vi "实验3 频率调制TX.vi"() -> ()   [LabVIEW 2015]
uses:
  <instrlib>/niUSRP/niUSRP Write Tx Data (CDB WDT).vi
panel:
  in  "同时播放？":bool
  out "错误":bool
  in  "FM频偏(Hz)":dbl=100000.0 format="%#_6p"
  in  "天线":string(combo)="TX1"
  in  "载波频率":dbl=800000000.0 format="%#_6p"
  in  "IQ 速率":dbl=400000.0 format="%#_6p"
  in  "增益":dbl format="%#_6f"
  in  "设备IP地址":refnum<k15>="192.168.10.2"
  out "FM调制信号(时域)":dbl[](graph) caption="FM 调制信号(时域)"
  out "FM调制信号(频域)":cluster{"f0":dbl, "df":dbl, "magnitude":dbl[]}(graph)={"f0"=-99993.30579988277, "df"=13.387776917911738, "magnitude"=[]}
  out "音频波形":waveform(dbl)(graph)={"t0"=timestamp(24.71655328798186 s since 1904-01-01), "dt"=2.2675736961451248e-05, "Y"=[]}
  in  "停止":bool
  in  "文件路径":path
  # "实验3 频率调制 TX"
  # "硬件参数配置"
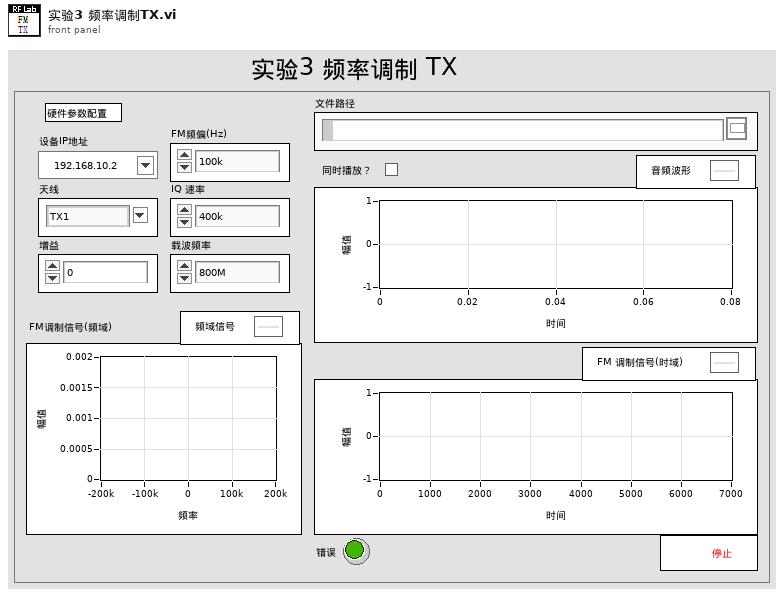
[diagram p1: front panel]
types:
  T1 = typedef "Sound Output Task ID.ctl" = u32
  T2 = typedef "Sound File Refnum.ctl" = refnum<file>
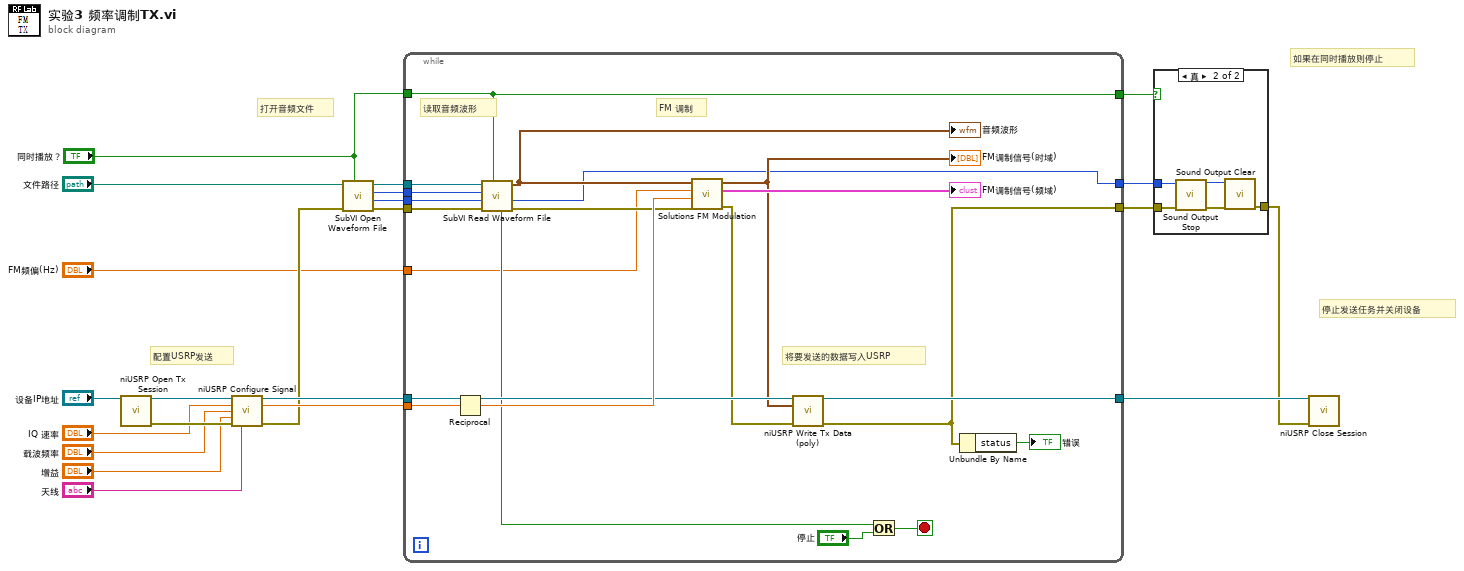
[diagram p0: block diagram]
diagram:
  # "停止发送任务并关闭设备"
  # "如果在同时播放则停止"
  # "配置USRP发送"
  # "打开音频文件"
  n1 = call <instrlib>:"niUSRP Open Tx Session.vi"("device names"="设备IP地址") -> ("session handle out"=w10:refnum<k15>, "error out"=w9:errorcluster)  [unwired: 13 in]
  n2 = call <instrlib>:"niUSRP Configure Signal.vi"("session handle"=w10, "IQ rate"="IQ 速率", "carrier frequency"="载波频率", "gain"="增益", "error in (no error)"=w9, "active antenna"="天线") -> ("session handle out"=w20:refnum<k15>, "coerced IQ rate"=w15:dbl, "error out"=w13:errorcluster)  [unwired: 5 in, 2 out]
  n3 = call "SubVI Open Waveform File.vi"("同时播放？"="同时播放？", "错误输入"=w13, "文件路径"="文件路径") -> ("错误输出"=w17:errorcluster, "音频输出任务ID"=w16:T1, "每通道采样数"=w14:i32, "声音文件引用句柄"=w21:T2)  [unwired: 5 in]
  n4 = while {
    tunnel: w21 -> [w43]
    tunnel: w17 -> [w42]
    tunnel: w15 -> [w40]
    tunnel: w20 -> [w39]
    tunnel: [w38] -> w3
    tunnel: [w25] -> w19
    tunnel: [w31] -> w18
    tunnel: w16 -> [w29]
    tunnel: w14 -> [w28]
    tunnel: "FM频偏(Hz)" -> [w26]
    tunnel: "同时播放？" -> [w23]
    tunnel: [w23] -> w1
    stop <- w37 stop-if-true
    # "将要发送的数据写入USRP"
    # "FM 调制"
    # "读取音频波形"
    n5 = Reciprocal(x=w40) -> (1/x=w41:dbl)
    n6 = call "SubVI Read Waveform File.vi"("同时播放？"=w23, "错误输入（无错误）"=w42, "音频输出任务ID"=w29, "每通道采样数"=w28, "声音文件引用句柄"=w43) -> ("错误输出"=w34:errorcluster, "音频输出任务ID"=w31:T1, "音频数据输出"=w35:waveform(dbl), "文件结束?"=w30:bool)  [unwired: 3 in]
    "音频波形" <- w35
    n7 = call "Solutions FM Modulation.vi"("错误输入(无错误)"=w34, "采样间隔(s)"=w41, "FM 频偏(Hz)"=w26, "数据输入"=w35) -> ("错误输出"=w27:errorcluster, "FM 调制信号(频域)"=→"FM调制信号(频域)":cluster{"f0":dbl, "df":dbl, "magnitude":dbl[]}, "FM 调制信号(时域)"=w32:waveform(cdb))  [unwired: 5 in]
    "FM调制信号(时域)" <- w32
    n8 = call-poly <instrlib>:"niUSRP Write Tx Data (poly).vi"("session handle"=w39, "data"=w32, "error in (no error)"=w27) -> ("session handle out"=w38:refnum<k15>, "error out"=w25:errorcluster)  [unwired: 11 in]
    n9 = Or(x=w30, y="停止") -> (x .or. y?=w37:bool)
    n10 = Unbundle By Name(w25) -> ("status"=→"错误":bool)
  }
  n11 = case shown="真" w1 {
    tunnel: w19 -> [w44 w49]
    tunnel: w18 -> [_ w48]
    tunnel: [w44 w45] -> w2
    frame False {
    }
    frame True {
      n12 = call <vilib>:"Sound Output Stop.vi"("error in (no error)"=w49, "task ID"=w48) -> ("error out"=w47:errorcluster, "task ID out"=w46:T1)  [unwired: 8 in]
      n13 = call <vilib>:"Sound Output Clear.vi"("error in (no error)"=w47, "task ID"=w46) -> ("error out"=w45:errorcluster)  [unwired: 9 in]
    }
  }
  n14 = call <instrlib>:"niUSRP Close Session.vi"("session handle"=w3, "error in (no error)"=w2) -> ()  [unwired: 13 in, 1 out]
